vi "Generate Circle Maps.vi"(6 "Auto Release Amount of Lines (Enabled)":bool=TRUE, 8 "error in (no error)":errorcluster, 11 "Amount of Lines":refnum<class "1D Array s32.lvclass">) -> (0 "error out":errorcluster, 1 "Keys":refnum<class "2D Array u32.lvclass">, 2 "Point mask within bounds":refnum<class "2D Array binary.lvclass">, 3 "Circle Scales":refnum<class "2D Array f32.lvclass">)   [LabVIEW 2020, in "G2CPU Line Profile.lvlib"]
uses:
  G2CPU Line Profile.lvlib
  <vilib>/Natan Biesmans/G2CPU GPU and CPU HPC Toolkit/G2CPU Libraries/Arrays/1DArray/s32/1D Array s32.lvclass
  C:/Program Files/National Instruments/LabVIEW 2025/vi.lib/Natan Biesmans/G2CPU GPU and CPU HPC Toolkit/G2CPU Libraries/Arrays/Array/Array Prototype.lvclass
  <vilib>/Natan Biesmans/G2CPU GPU and CPU HPC Toolkit/G2CPU Libraries/Arrays/2DArray/binary/2D Array binary.lvclass
  <vilib>/Natan Biesmans/G2CPU GPU and CPU HPC Toolkit/G2CPU Libraries/Arrays/2DArray/u32/2D Array u32.lvclass
  <vilib>/Natan Biesmans/G2CPU GPU and CPU HPC Toolkit/G2CPU Libraries/Arrays/2DArray/f32/2D Array f32.lvclass
  <vilib>/Natan Biesmans/G2CPU GPU and CPU HPC Toolkit/G2CPU Libraries/Arrays/Array/Array Prototype.lvclass/Array Prototype.ctl
  f10c7694-f2bd-4e2a-b4ac-6f0ce56305b5.vi
  c325dd27-5db5-468d-a647-380cace1f88b.vi
  4e0a4381-b441-4684-99d3-9e292b538594.vi
  6d135c47-d03c-422a-b192-5cccd0943e62.vi
  3bccb9bb-66c2-4dbf-b486-1666d0f23caa.vi
  88953b0a-fa42-4f47-9fbe-798db8d0607b.vi
  d2b44248-1ab6-419b-8898-c4fe5bd77a59.vi
  bd523468-f17e-4d84-9a98-c6a5fbe0f2c3.vi
  4f08f1e8-1ded-4970-9208-753e27e1f13d.vi
  <vilib>/Natan Biesmans/G2CPU GPU and CPU HPC Toolkit/G2CPU Libraries/Arrays/Array/G2CPU Get Array Pointer.vi
  f10c7694-f2bd-4e2a-b4ac-6f0ce56305b5.vi/72eb0651-ae32-4ba2-a447-070823507cb2.vi
  c325dd27-5db5-468d-a647-380cace1f88b.vi/e7247370-a01f-465a-ac0e-4dfefcb1bb87.vi
  c325dd27-5db5-468d-a647-380cace1f88b.vi/345e91f0-9a5e-4de4-af9c-133346717e4a.vi
  4e0a4381-b441-4684-99d3-9e292b538594.vi/ab6cfe59-c8ad-4da3-839b-8d02ec9e015f.vi
  6d135c47-d03c-422a-b192-5cccd0943e62.vi/ab6cfe59-c8ad-4da3-839b-8d02ec9e015f.vi
  3bccb9bb-66c2-4dbf-b486-1666d0f23caa.vi/cfed8f62-9c64-4dab-912e-5e7c21cb720b.vi
  88953b0a-fa42-4f47-9fbe-798db8d0607b.vi/5793b77b-c002-4ebf-9075-685617c95341.vi
  88953b0a-fa42-4f47-9fbe-798db8d0607b.vi/2ed3ef86-c00d-4d71-b84c-20267a6dfcf9.vi
  d2b44248-1ab6-419b-8898-c4fe5bd77a59.vi/2cbae9c5-d993-4013-91e6-67de96abb5a0.vi
  d2b44248-1ab6-419b-8898-c4fe5bd77a59.vi/df7b902d-6356-419a-b5d5-2ac54df1e506.vi
  bd523468-f17e-4d84-9a98-c6a5fbe0f2c3.vi/46771f49-eb1d-473b-8e81-f516cef50a4e.vi
  bd523468-f17e-4d84-9a98-c6a5fbe0f2c3.vi/dc76f8e4-64fa-456a-8549-7a4b6936c4c9.vi
  bd523468-f17e-4d84-9a98-c6a5fbe0f2c3.vi/7e60ddfb-e748-4c0c-85da-e395a1b7978d.vi
  bd523468-f17e-4d84-9a98-c6a5fbe0f2c3.vi/d2eceff7-f641-4ce4-acfa-e9e293a3c877.vi
  bd523468-f17e-4d84-9a98-c6a5fbe0f2c3.vi/b737122b-4036-448b-abd3-e2701355e828.vi
  4f08f1e8-1ded-4970-9208-753e27e1f13d.vi/6197f869-f6d4-49b3-9b2c-cc979b422c2e.vi
  4f08f1e8-1ded-4970-9208-753e27e1f13d.vi/a7e86dbb-b4c0-485c-89c5-522e60ee265c.vi
  4e0a4381-b441-4684-99d3-9e292b538594.vi/ab6cfe59-c8ad-4da3-839b-8d02ec9e015f.vi/313ec8c5-c203-475c-9de0-0583f6fb8b4d.vi
  6d135c47-d03c-422a-b192-5cccd0943e62.vi/ab6cfe59-c8ad-4da3-839b-8d02ec9e015f.vi/313ec8c5-c203-475c-9de0-0583f6fb8b4d.vi
  3bccb9bb-66c2-4dbf-b486-1666d0f23caa.vi/cfed8f62-9c64-4dab-912e-5e7c21cb720b.vi/77c7badc-ed81-4514-99c1-20d37f4e5ecc.vi
  3bccb9bb-66c2-4dbf-b486-1666d0f23caa.vi/cfed8f62-9c64-4dab-912e-5e7c21cb720b.vi/eb76fa01-6782-47b4-b34f-9eb474c9cc78.vi
  <vilib>/Natan Biesmans/G2CPU GPU and CPU HPC Toolkit/ArrayFire Driver/VIs/Run as Multi Device.vi
  88953b0a-fa42-4f47-9fbe-798db8d0607b.vi/5793b77b-c002-4ebf-9075-685617c95341.vi/3e802c67-fb96-46a3-ae13-4994a8508b4f.vi
  88953b0a-fa42-4f47-9fbe-798db8d0607b.vi/5793b77b-c002-4ebf-9075-685617c95341.vi/5a50fc67-79e7-4972-80c2-92243cd53dd4.vi
  88953b0a-fa42-4f47-9fbe-798db8d0607b.vi/2ed3ef86-c00d-4d71-b84c-20267a6dfcf9.vi/730f6c57-5c0b-4ee9-b61e-75067b25222b.vi
  88953b0a-fa42-4f47-9fbe-798db8d0607b.vi/2ed3ef86-c00d-4d71-b84c-20267a6dfcf9.vi/096b8799-7810-404e-baca-ba9279cec4bd.vi
  88953b0a-fa42-4f47-9fbe-798db8d0607b.vi/2ed3ef86-c00d-4d71-b84c-20267a6dfcf9.vi/0f1a5a47-bcc5-4796-ac31-8dfcfbc0d7d1.vi
  88953b0a-fa42-4f47-9fbe-798db8d0607b.vi/2ed3ef86-c00d-4d71-b84c-20267a6dfcf9.vi/89f12e17-3330-4b72-ad8f-8dd636660732.vi
  d2b44248-1ab6-419b-8898-c4fe5bd77a59.vi/df7b902d-6356-419a-b5d5-2ac54df1e506.vi/edd31282-7992-4bba-af75-482693dee5e1.vi
  bd523468-f17e-4d84-9a98-c6a5fbe0f2c3.vi/dc76f8e4-64fa-456a-8549-7a4b6936c4c9.vi/3e802c67-fb96-46a3-ae13-4994a8508b4f.vi
  bd523468-f17e-4d84-9a98-c6a5fbe0f2c3.vi/dc76f8e4-64fa-456a-8549-7a4b6936c4c9.vi/5a50fc67-79e7-4972-80c2-92243cd53dd4.vi
  bd523468-f17e-4d84-9a98-c6a5fbe0f2c3.vi/dc76f8e4-64fa-456a-8549-7a4b6936c4c9.vi/1c928fc9-710a-40e7-8c4f-08a1069452ae.vi
  4f08f1e8-1ded-4970-9208-753e27e1f13d.vi/6197f869-f6d4-49b3-9b2c-cc979b422c2e.vi/3e802c67-fb96-46a3-ae13-4994a8508b4f.vi
  4f08f1e8-1ded-4970-9208-753e27e1f13d.vi/6197f869-f6d4-49b3-9b2c-cc979b422c2e.vi/5a50fc67-79e7-4972-80c2-92243cd53dd4.vi
  4f08f1e8-1ded-4970-9208-753e27e1f13d.vi/a7e86dbb-b4c0-485c-89c5-522e60ee265c.vi/730f6c57-5c0b-4ee9-b61e-75067b25222b.vi
  4f08f1e8-1ded-4970-9208-753e27e1f13d.vi/a7e86dbb-b4c0-485c-89c5-522e60ee265c.vi/096b8799-7810-404e-baca-ba9279cec4bd.vi
  4f08f1e8-1ded-4970-9208-753e27e1f13d.vi/a7e86dbb-b4c0-485c-89c5-522e60ee265c.vi/0f1a5a47-bcc5-4796-ac31-8dfcfbc0d7d1.vi
  4f08f1e8-1ded-4970-9208-753e27e1f13d.vi/a7e86dbb-b4c0-485c-89c5-522e60ee265c.vi/89f12e17-3330-4b72-ad8f-8dd636660732.vi
  bd523468-f17e-4d84-9a98-c6a5fbe0f2c3.vi/dc76f8e4-64fa-456a-8549-7a4b6936c4c9.vi/3e802c67-fb96-46a3-ae13-4994a8508b4f.vi/1b7cf390-2ae0-48f3-9bce-03c57eed6ee8.vi
  4f08f1e8-1ded-4970-9208-753e27e1f13d.vi/a7e86dbb-b4c0-485c-89c5-522e60ee265c.vi/730f6c57-5c0b-4ee9-b61e-75067b25222b.vi/0070e0fe-4ad7-4a3e-8965-d64becb7e5f0.vi
  <vilib>/Natan Biesmans/G2CPU GPU and CPU HPC Toolkit/G2CPU Libraries/Arrays/1DArray/f32/1D Array f32.lvclass
  <vilib>/Natan Biesmans/G2CPU GPU and CPU HPC Toolkit/ArrayFire Driver/VIs/max all.vi
  <vilib>/Natan Biesmans/G2CPU GPU and CPU HPC Toolkit/G2CPU Libraries/Arrays/Array/G2CPU Release Array.vi
  <vilib>/Natan Biesmans/G2CPU GPU and CPU HPC Toolkit/ArrayFire Driver/VIs/cast.vi
  <vilib>/Natan Biesmans/G2CPU GPU and CPU HPC Toolkit/G2CPU Libraries/Arrays/Array/G2CPU Set Array Pointer.vi
  <vilib>/Natan Biesmans/G2CPU GPU and CPU HPC Toolkit/ArrayFire Driver/VIs/range.vi
  <vilib>/Natan Biesmans/G2CPU GPU and CPU HPC Toolkit/ArrayFire Driver/VIs/iszero.vi
  <vilib>/Natan Biesmans/G2CPU GPU and CPU HPC Toolkit/ArrayFire Driver/VIs/sub.vi
  <vilib>/Natan Biesmans/G2CPU GPU and CPU HPC Toolkit/ArrayFire Driver/VIs/release array.vi
  <vilib>/Natan Biesmans/G2CPU GPU and CPU HPC Toolkit/ArrayFire Driver/subvi/Error Converter (ErrCode or Status).vi
  <vilib>/Natan Biesmans/G2CPU GPU and CPU HPC Toolkit/ArrayFire Driver/VIs/add.vi
  <vilib>/Natan Biesmans/G2CPU GPU and CPU HPC Toolkit/G2CPU Libraries/Arrays/SubVI/is 2D.vi
  <vilib>/Natan Biesmans/G2CPU GPU and CPU HPC Toolkit/ArrayFire Driver/VIs/lt.vi
  <vilib>/Natan Biesmans/G2CPU GPU and CPU HPC Toolkit/G2CPU Libraries/Arrays/SubVI/is 1D.vi
  <vilib>/Natan Biesmans/G2CPU GPU and CPU HPC Toolkit/ArrayFire Driver/VIs/div.vi
  <vilib>/Natan Biesmans/G2CPU GPU and CPU HPC Toolkit/ArrayFire Driver/VIs/mul.vi
  <vilib>/Natan Biesmans/G2CPU GPU and CPU HPC Toolkit/G2CPU Libraries/Arrays/Array/Array Prototype.lvclass
  <vilib>/Natan Biesmans/G2CPU GPU and CPU HPC Toolkit/G2CPU Libraries/Arrays/1DArray/1D Array Prototype.lvclass
  <vilib>/Natan Biesmans/G2CPU GPU and CPU HPC Toolkit/G2CPU Libraries/Arrays/2DArray/2D Array Prototype.lvclass
  <vilib>/Natan Biesmans/G2CPU GPU and CPU HPC Toolkit/G2CPU Libraries/Arrays/DataTypes/f32/f32.lvclass
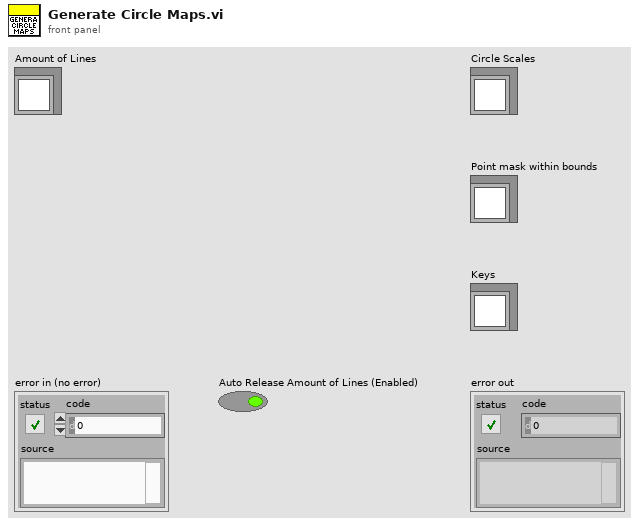
[diagram p1: front panel]
types:
  T1 = typedef "AF.lvlib/Dim4.ctl" = cluster{"Dim 0":u64, "Dim 1":u64, "Dim 2":u64, "Dim 3":u64}
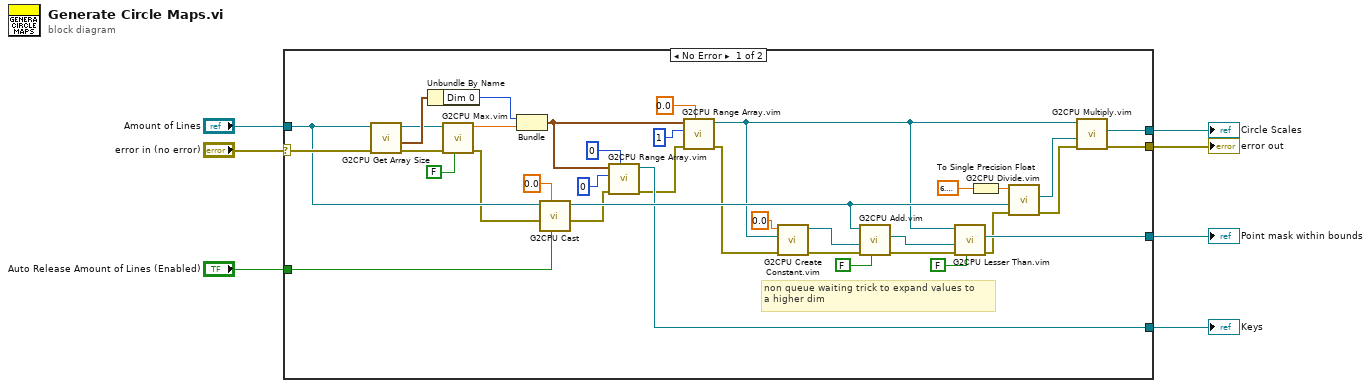
[diagram p0: block diagram]
diagram:
  n1 = case shown="No Error" "error in (no error)" {
    selector: "error in (no error)" -> [w44 w45]
    tunnel: "Amount of Lines" -> [w43 _]
    tunnel: [w42 _] -> w5
    tunnel: [w27 _] -> w4
    tunnel: [w14 _] -> w3
    tunnel: [w13 w45] -> w2
    tunnel: "Auto Release Amount of Lines (Enabled)" -> [w8 _]
    frame No Error {
      # "non queue waiting trick to expand values to\na higher dim"
      n2 = call <vilib>:"G2CPU Get Array Size.vi"("error in (no error)"=w44, "Array in"=w43) -> ("error out"=w30:errorcluster, "Array Size"=w31:T1, "Array out"=w29:refnum<class "1D Array s32.lvclass">)  [unwired: 6 in, 1 out]
      n3 = Unbundle By Name(w31) -> ("Dim 0"=w11:u64)
      n4 = call "G2CPU Max.vim"("Auto Release (Enabled)"=FALSE, "error in (no error)"=w30, "Array First"=w29) -> ("error out"=w19:errorcluster, "real out"=w15:dbl)  [unwired: 6 in, 1 out]
      n5 = Bundle("Dim 0"=w11, "real out"=w15) -> (w24:cluster{"Dim 0":u64, "real out":dbl})  [unwired: 1 in]
      n6 = call "G2CPU Cast"("Auto Release Low (Enabled)"=w8, "Datatype Prototype"=sgl 0.0 ("single precision float"), "error in (no error)"=w19, "Array In"=w43) -> ("error out"=w25:errorcluster, "Array Out"=w38:refnum<class "1D Array f32.lvclass">)  [unwired: 6 in]
      n7 = call "G2CPU Range Array.vim"("Datatype"=u32 0, "Error in"=w25, "Sequential Dimension"=0, "Size"=w24) -> ("error out"=w26:errorcluster, "Array out"=w27:refnum<class "2D Array u32.lvclass">)  [unwired: 6 in]
      n8 = call "G2CPU Range Array.vim"("Datatype"=sgl 0.0, "Error in"=w26, "Sequential Dimension"=1, "Size"=w24) -> ("error out"=w33:errorcluster, "Array out"=w34:refnum<class "2D Array f32.lvclass">)  [unwired: 6 in]
      n9 = call "G2CPU Create Constant.vim"("error in (no error)"=w33, "Size"=w34, "val"=sgl 0.0) -> ("error out"=w35:errorcluster, "object out"=w37:refnum<class "2D Array f32.lvclass">)  [unwired: 7 in]
      n10 = call "G2CPU Add.vim"("Auto Release lhs (Enabled)"=FALSE, "error in (no error)"=w35, "Array rhs"=w37, "Array lhs"=w38) -> ("error out"=w36:errorcluster, "Array Result"=w39:refnum<class "2D Array f32.lvclass">)  [unwired: 6 in]
      n11 = call "G2CPU Lesser Than.vim"("Auto Release lhs (Enabled)"=FALSE, "error in (no error)"=w36, "Array rhs"=w39, "Array lhs"=w34) -> ("error out"=w28:errorcluster, "Array Result"=w42:refnum<class "2D Array binary.lvclass">)  [unwired: 6 in]
      n12 = To Single Precision Float(number=6.283185307179586) -> (single precision float=w21:sgl)
      n13 = call "G2CPU Divide.vim"("error in (no error)"=w28, "Array rhs"=w38, "Array lhs"=w21) -> ("error out"=w17:errorcluster, "Array Result"=w20:refnum<class "1D Array f32.lvclass">)  [unwired: 7 in]
      n14 = call "G2CPU Multiply.vim"("error in (no error)"=w17, "Array rhs"=w20, "Array lhs"=w34) -> ("error out"=w13:errorcluster, "Array Result"=w14:refnum<class "2D Array f32.lvclass">)  [unwired: 7 in]
    }
    frame Error {
    }
  }
  "Point mask within bounds" <- w5
  "Keys" <- w4
  "Circle Scales" <- w3
  "error out" <- w2
